vi "_old_Load_SetList_v4.10_DDS.vi"(0 "Path":path) -> (1 "Procedure Name":string="IBS_PICameraTest_29Sep04", 2 "Paramaters":T2={"Master PB Staging List"=[{"Output Bits"=[], "Delay (s)"="", "String"="", "Halt?"=FALSE}, {"Output Bits"=[], "Delay (s)"="", "String"="", "Halt?"=FALSE}, {"Output Bits"=[], "Delay (s)"="", "String"="", "Halt?"=FALSE}, {"Output Bits"=[], "Delay (s)"="", "String"="", "Halt?"=FALSE}, {"Output Bits"=[], "Delay (s)"="", "String"="", "Halt?"=FALSE}, {"Output Bits"=[], "Delay (s)"="", "String"="", "Halt?"=FALSE}, {"Output Bits"=[], "Delay (s)"="", "String"="", "Halt?"=FALSE}, {"Output Bits"=[], "Delay (s)"="", "String"="", "Halt?"=FALSE}, {"Output Bits"=[], "Delay (s)"="", "String"="", "Halt?"=FALSE}, {"Output Bits"=[], "Delay (s)"="", "String"="", "Halt?"=FALSE}, {"Output Bits"=[], "Delay (s)"="", "String"="", "Halt?"=FALSE}, {"Output Bits"=[], "Delay (s)"="", "String"="", "Halt?"=FALSE}, {"Output Bits"=[], "Delay (s)"="", "String"="", "Halt?"=FALSE}, {"Output Bits"=[], "Delay (s)"="", "String"="", "Halt?"=FALSE}, {"Output Bits"=[], "Delay (s)"="", "String"="", "Halt?"=FALSE}, {"Output Bits"=[], "Delay (s)"="", "String"="", "Halt?"=FALSE}, {"Output Bits"=[], "Delay (s)"="", "String"="", "Halt?"=FALSE}, {"Output Bits"=[], "Delay (s)"="", "String"="", "Halt?"=FALSE}, {"Output Bits"=[], "Delay (s)"="", "String"="", "Halt?"=FALSE}, {"Output Bits"=[], "Delay (s)"="", "String"="", "Halt?"=FALSE}, {"Output Bits"=[], "Delay (s)"="", "String"="", "Halt?"=FALSE}, {"Output Bits"=[], "Delay (s)"="", "String"="", "Halt?"=FALSE}, {"Output Bits"=[], "Delay (s)"="", "String"="", "Halt?"=FALSE}, {"Output Bits"=[], "Delay (s)"="", "String"="", "Halt?"=FALSE}, {"Output Bits"=[], "Delay (s)"="", "String"="", "Halt?"=FALSE}, {"Output Bits"=[], "Delay (s)"="", "String"="", "Halt?"=FALSE}, {"Output Bits"=[], "Delay (s)"="", "String"="", "Halt?"=FALSE}, {"Output Bits"=[], "Delay (s)"="", "String"="", "Halt?"=FALSE}, {"Output Bits"=[], "Delay (s)"="", "String"="", "Halt?"=FALSE}, {"Output Bits"=[], "Delay (s)"="", "String"="", "Halt?"=FALSE}, {"Output Bits"=[], "Delay (s)"="", "String"="", "Halt?"=FALSE}, {"Output Bits"=[], "Delay (s)"="", "String"="", "Halt?"=FALSE}, {"Output Bits"=[], "Delay (s)"="", "String"="", "Halt?"=FALSE}, {"Output Bits"=[], "Delay (s)"="", "String"="", "Halt?"=FALSE}, {"Output Bits"=[], "Delay (s)"="", "String"="", "Halt?"=FALSE}, {"Output Bits"=[], "Delay (s)"="", "String"="", "Halt?"=FALSE}, {"Output Bits"=[], "Delay (s)"="", "String"="", "Halt?"=FALSE}, {"Output Bits"=[], "Delay (s)"="", "String"="", "Halt?"=FALSE}, {"Output Bits"=[], "Delay (s)"="", "String"="", "Halt?"=FALSE}, {"Output Bits"=[], "Delay (s)"="", "String"="", "Halt?"=FALSE}, {"Output Bits"=[], "Delay (s)"="", "String"="", "Halt?"=FALSE}, {"Output Bits"=[], "Delay (s)"="", "String"="", "Halt?"=FALSE}, {"Output Bits"=[], "Delay (s)"="", "String"="", "Halt?"=FALSE}, {"Output Bits"=[], "Delay (s)"="", "String"="", "Halt?"=FALSE}], "Slave PB Staging List"=[{"Output Bits"=[], "Delay (s)"="", "String"="", "Halt?"=FALSE}, {"Output Bits"=[], "Delay (s)"="", "String"="", "Halt?"=FALSE}, {"Output Bits"=[], "Delay (s)"="", "String"="", "Halt?"=FALSE}, {"Output Bits"=[], "Delay (s)"="", "String"="", "Halt?"=FALSE}, {"Output Bits"=[], "Delay (s)"="", "String"="", "Halt?"=FALSE}, {"Output Bits"=[], "Delay (s)"="", "String"="", "Halt?"=FALSE}, {"Output Bits"=[], "Delay (s)"="", "String"="", "Halt?"=FALSE}, {"Output Bits"=[], "Delay (s)"="", "String"="", "Halt?"=FALSE}, {"Output Bits"=[], "Delay (s)"="", "String"="", "Halt?"=FALSE}, {"Output Bits"=[], "Delay (s)"="", "String"="", "Halt?"=FALSE}, {"Output Bits"=[], "Delay (s)"="", "String"="", "Halt?"=FALSE}, {"Output Bits"=[], "Delay (s)"="", "String"="", "Halt?"=FALSE}, {"Output Bits"=[], "Delay (s)"="", "String"="", "Halt?"=FALSE}, {"Output Bits"=[], "Delay (s)"="", "String"="", "Halt?"=FALSE}, {"Output Bits"=[], "Delay (s)"="", "String"="", "Halt?"=FALSE}, {"Output Bits"=[], "Delay (s)"="", "String"="", "Halt?"=FALSE}, {"Output Bits"=[], "Delay (s)"="", "String"="", "Halt?"=FALSE}, {"Output Bits"=[], "Delay (s)"="", "String"="", "Halt?"=FALSE}, {"Output Bits"=[], "Delay (s)"="", "String"="", "Halt?"=FALSE}, {"Output Bits"=[], "Delay (s)"="", "String"="", "Halt?"=FALSE}, {"Output Bits"=[], "Delay (s)"="", "String"="", "Halt?"=FALSE}, {"Output Bits"=[], "Delay (s)"="", "String"="", "Halt?"=FALSE}, {"Output Bits"=[], "Delay (s)"="", "String"="", "Halt?"=FALSE}, {"Output Bits"=[], "Delay (s)"="", "String"="", "Halt?"=FALSE}, {"Output Bits"=[], "Delay (s)"="", "String"="", "Halt?"=FALSE}, {"Output Bits"=[], "Delay (s)"="", "String"="", "Halt?"=FALSE}, {"Output Bits"=[], "Delay (s)"="", "String"="", "Halt?"=FALSE}, {"Output Bits"=[], "Delay (s)"="", "String"="", "Halt?"=FALSE}, {"Output Bits"=[], "Delay (s)"="", "String"="", "Halt?"=FALSE}, {"Output Bits"=[], "Delay (s)"="", "String"="", "Halt?"=FALSE}, {"Output Bits"=[], "Delay (s)"="", "String"="", "Halt?"=FALSE}, {"Output Bits"=[], "Delay (s)"="", "String"="", "Halt?"=FALSE}, {"Output Bits"=[], "Delay (s)"="", "String"="", "Halt?"=FALSE}, {"Output Bits"=[], "Delay (s)"="", "String"="", "Halt?"=FALSE}, {"Output Bits"=[], "Delay (s)"="", "String"="", "Halt?"=FALSE}, {"Output Bits"=[], "Delay (s)"="", "String"="", "Halt?"=FALSE}, {"Output Bits"=[], "Delay (s)"="", "String"="", "Halt?"=FALSE}, {"Output Bits"=[], "Delay (s)"="", "String"="", "Halt?"=FALSE}, {"Output Bits"=[], "Delay (s)"="", "String"="", "Halt?"=FALSE}, {"Output Bits"=[], "Delay (s)"="", "String"="", "Halt?"=FALSE}, {"Output Bits"=[], "Delay (s)"="", "String"="", "Halt?"=FALSE}, {"Output Bits"=[], "Delay (s)"="", "String"="", "Halt?"=FALSE}, {"Output Bits"=[], "Delay (s)"="", "String"="", "Halt?"=FALSE}, {"Output Bits"=[], "Delay (s)"="", "String"="", "Halt?"=FALSE}], "Novatech Ramps"=[{"Ramp Channels"=[], "2 Freq. [MHz]"="", "2 Power [dBm]"="", "3 Freq. [MHz]"="", "3 Power [dBm]"="", "Serial Port"=""}, {"Ramp Channels"=[], "2 Freq. [MHz]"="", "2 Power [dBm]"="", "3 Freq. [MHz]"="", "3 Power [dBm]"="", "Serial Port"=""}, {"Ramp Channels"=[], "2 Freq. [MHz]"="", "2 Power [dBm]"="", "3 Freq. [MHz]"="", "3 Power [dBm]"="", "Serial Port"=""}, {"Ramp Channels"=[], "2 Freq. [MHz]"="", "2 Power [dBm]"="", "3 Freq. [MHz]"="", "3 Power [dBm]"="", "Serial Port"=""}, {"Ramp Channels"=[], "2 Freq. [MHz]"="", "2 Power [dBm]"="", "3 Freq. [MHz]"="", "3 Power [dBm]"="", "Serial Port"=""}, {"Ramp Channels"=[], "2 Freq. [MHz]"="", "2 Power [dBm]"="", "3 Freq. [MHz]"="", "3 Power [dBm]"="", "Serial Port"=""}, {"Ramp Channels"=[], "2 Freq. [MHz]"="", "2 Power [dBm]"="", "3 Freq. [MHz]"="", "3 Power [dBm]"="", "Serial Port"=""}], "Sequencing Info"=[{"Start"=0.0, "End"=2.11, "Sequenced Data"=[], "Inform\nIgor?"=FALSE, "Computed Step Size"=0.0, "Procedure Variable"="", "Default"=2.11, "Steps"=0}], "SRS Ramps"=[{"lattice ramp"=[{"dt"="", "formula"=""}, {"dt"="", "formula"=""}, {"dt"="", "formula"=""}], "Output"=[{"Time Values"=[0.0, 0.002, 0.004, 0.006, 0.008, 0.01, 0.012, 0.014, 0.016, 0.018000000000000002, 0.02, 0.022, 0.024, 0.026000000000000002, 0.028, 0.03, 0.032, 0.034, 0.036000000000000004, 0.038, 0.04, 0.042, 0.044, 0.046, 0.048, 0.05, 0.052000000000000005, 0.054, 0.056, 0.058, 0.06, 0.062, 0.064, 0.066, 0.068, 0.07, 0.07200000000000001, 0.074, 0.076, 0.078, 0.08, 0.082, 0.084, 0.08600000000000001, 0.088, 0.09, 0.092, 0.094, 0.096, 0.098, 0.1, 0.10200000000000001, 0.10400000000000001, 0.106, 0.108, 0.11, 0.112, 0.114, 0.116, 0.11800000000000001, 0.12, 0.122, 0.124, 0.126, 0.128, 0.13, 0.132, 0.134, 0.136, 0.138, 0.14, 0.14200000000000002, 0.14400000000000002, 0.146, 0.148, 0.15, 0.152, 0.154, 0.156, 0.158, 0.16, 0.162, 0.164, 0.166, 0.168, 0.17, 0.17200000000000001, 0.17400000000000002, 0.176, 0.178, 0.18, 0.182, 0.184, 0.186, 0.188, 0.19, 0.192, 0.194, 0.196, 0.198, 0.2, 0.6000000000000001, 0.6000000000000001, 0.6002000000000001, 0.6004, 0.6006000000000001, 0.6008000000000001, 0.6010000000000001, 0.6012000000000001, 0.6014, 0.6016000000000001, 0.6018000000000001, 0.6020000000000001, 0.6022000000000001, 0.6024, 0.6026000000000001, 0.6028000000000001, 0.6030000000000001, 0.6032000000000001, 0.6034, 0.6036000000000001, 0.6038000000000001, 0.6040000000000001, 0.6042000000000001, 0.6044, 0.6046000000000001, 0.6048000000000001, 0.6050000000000001, 0.6052000000000001, 0.6054, 0.6056000000000001, 0.6058000000000001, 0.6060000000000001, 0.6062000000000001, 0.6064, 0.6066000000000001, 0.6068000000000001, 0.6070000000000001, 0.6072000000000001, 0.6074, 0.6076000000000001, 0.6078000000000001, 0.6080000000000001, 0.6082000000000001, 0.6084, 0.6086000000000001, 0.6088000000000001, 0.6090000000000001, 0.6092000000000001, 0.6094, 0.6096000000000001, 0.6098000000000001, 0.6100000000000001, 0.6102000000000001, 0.6104, 0.6106000000000001, 0.6108000000000001, 0.6110000000000001, 0.6112000000000001, 0.6114, 0.6116000000000001, 0.6118000000000001, 0.6120000000000001, 0.6122000000000001, 0.6124, 0.6126, 0.6128000000000001, 0.6130000000000001, 0.6132000000000001, 0.6134000000000001, 0.6136000000000001, 0.6138000000000001, 0.6140000000000001, 0.6142000000000001, 0.6144000000000001, 0.6146, 0.6148000000000001, 0.6150000000000001, 0.6152000000000001, 0.6154000000000001, 0.6156, 0.6158000000000001, 0.6160000000000001, 0.6162000000000001, 0.6164000000000001, 0.6166, 0.6168000000000001, 0.6170000000000001, 0.6172000000000001, 0.6174000000000001, 0.6176, 0.6178000000000001, 0.6180000000000001, 0.6182000000000001, 0.6184000000000001, 0.6186, 0.6188000000000001, 0.6190000000000001, 0.6192000000000001, 0.6194000000000001, 0.6196, 0.6198000000000001, 0.6200000000000001, 0.6202000000000001, 0.6212000000000001], array[205 elements]}, {"Time Values"=[0.0, 0.002, 0.004, 0.006, 0.008, 0.01, 0.012, 0.014, 0.016, 0.018000000000000002, 0.02, 0.022, 0.024, 0.026000000000000002, 0.028, 0.03, 0.032, 0.034, 0.036000000000000004, 0.038, 0.04, 0.042, 0.044, 0.046, 0.048, 0.05, 0.052000000000000005, 0.054, 0.056, 0.058, 0.06, 0.062, 0.064, 0.066, 0.068, 0.07, 0.07200000000000001, 0.074, 0.076, 0.078, 0.08, 0.082, 0.084, 0.08600000000000001, 0.088, 0.09, 0.092, 0.094, 0.096, 0.098, 0.1, 0.10200000000000001, 0.10400000000000001, 0.106, 0.108, 0.11, 0.112, 0.114, 0.116, 0.11800000000000001, 0.12, 0.122, 0.124, 0.126, 0.128, 0.13, 0.132, 0.134, 0.136, 0.138, 0.14, 0.14200000000000002, 0.14400000000000002, 0.146, 0.148, 0.15, 0.152, 0.154, 0.156, 0.158, 0.16, 0.162, 0.164, 0.166, 0.168, 0.17, 0.17200000000000001, 0.17400000000000002, 0.176, 0.178, 0.18, 0.182, 0.184, 0.186, 0.188, 0.19, 0.192, 0.194, 0.196, 0.198, 0.2, 0.6000000000000001, 0.6000000000000001, 0.6002000000000001, 0.6004, 0.6006000000000001, 0.6008000000000001, 0.6010000000000001, 0.6012000000000001, 0.6014, 0.6016000000000001, 0.6018000000000001, 0.6020000000000001, 0.6022000000000001, 0.6024, 0.6026000000000001, 0.6028000000000001, 0.6030000000000001, 0.6032000000000001, 0.6034, 0.6036000000000001, 0.6038000000000001, 0.6040000000000001, 0.6042000000000001, 0.6044, 0.6046000000000001, 0.6048000000000001, 0.6050000000000001, 0.6052000000000001, 0.6054, 0.6056000000000001, 0.6058000000000001, 0.6060000000000001, 0.6062000000000001, 0.6064, 0.6066000000000001, 0.6068000000000001, 0.6070000000000001, 0.6072000000000001, 0.6074, 0.6076000000000001, 0.6078000000000001, 0.6080000000000001, 0.6082000000000001, 0.6084, 0.6086000000000001, 0.6088000000000001, 0.6090000000000001, 0.6092000000000001, 0.6094, 0.6096000000000001, 0.6098000000000001, 0.6100000000000001, 0.6102000000000001, 0.6104, 0.6106000000000001, 0.6108000000000001, 0.6110000000000001, 0.6112000000000001, 0.6114, 0.6116000000000001, 0.6118000000000001, 0.6120000000000001, 0.6122000000000001, 0.6124, 0.6126, 0.6128000000000001, 0.6130000000000001, 0.6132000000000001, 0.6134000000000001, 0.6136000000000001, 0.6138000000000001, 0.6140000000000001, 0.6142000000000001, 0.6144000000000001, 0.6146, 0.6148000000000001, 0.6150000000000001, 0.6152000000000001, 0.6154000000000001, 0.6156, 0.6158000000000001, 0.6160000000000001, 0.6162000000000001, 0.6164000000000001, 0.6166, 0.6168000000000001, 0.6170000000000001, 0.6172000000000001, 0.6174000000000001, 0.6176, 0.6178000000000001, 0.6180000000000001, 0.6182000000000001, 0.6184000000000001, 0.6186, 0.6188000000000001, 0.6190000000000001, 0.6192000000000001, 0.6194000000000001, 0.6196, 0.6198000000000001, 0.6200000000000001, 0.6202000000000001, 0.6212000000000001], array[205 elements]}], "SRS Selection"=enum."1550 Vertical"}, {"lattice ramp"=[{"dt"="", "formula"=""}], "Output"=[{"Time Values"=[0.0, 0.002, 0.004, 0.006, 0.008, 0.01, 0.012, 0.014, 0.016, 0.018000000000000002, 0.02, 0.022, 0.024, 0.026000000000000002, 0.028, 0.03, 0.032, 0.034, 0.036000000000000004, 0.038, 0.04, 0.042, 0.044, 0.046, 0.048, 0.05, 0.052000000000000005, 0.054, 0.056, 0.058, 0.06, 0.062, 0.064, 0.066, 0.068, 0.07, 0.07200000000000001, 0.074, 0.076, 0.078, 0.08, 0.082, 0.084, 0.08600000000000001, 0.088, 0.09, 0.092, 0.094, 0.096, 0.098, 0.1, 0.10200000000000001, 0.10400000000000001, 0.106, 0.108, 0.11, 0.112, 0.114, 0.116, 0.11800000000000001, 0.12, 0.122, 0.124, 0.126, 0.128, 0.13, 0.132, 0.134, 0.136, 0.138, 0.14, 0.14200000000000002, 0.14400000000000002, 0.146, 0.148, 0.15, 0.152, 0.154, 0.156, 0.158, 0.16, 0.162, 0.164, 0.166, 0.168, 0.17, 0.17200000000000001, 0.17400000000000002, 0.176, 0.178, 0.18, 0.182, 0.184, 0.186, 0.188, 0.19, 0.192, 0.194, 0.196, 0.198, 0.2, 0.6000000000000001, 0.6000000000000001, 0.6002000000000001, 0.6004, 0.6006000000000001, 0.6008000000000001, 0.6010000000000001, 0.6012000000000001, 0.6014, 0.6016000000000001, 0.6018000000000001, 0.6020000000000001, 0.6022000000000001, 0.6024, 0.6026000000000001, 0.6028000000000001, 0.6030000000000001, 0.6032000000000001, 0.6034, 0.6036000000000001, 0.6038000000000001, 0.6040000000000001, 0.6042000000000001, 0.6044, 0.6046000000000001, 0.6048000000000001, 0.6050000000000001, 0.6052000000000001, 0.6054, 0.6056000000000001, 0.6058000000000001, 0.6060000000000001, 0.6062000000000001, 0.6064, 0.6066000000000001, 0.6068000000000001, 0.6070000000000001, 0.6072000000000001, 0.6074, 0.6076000000000001, 0.6078000000000001, 0.6080000000000001, 0.6082000000000001, 0.6084, 0.6086000000000001, 0.6088000000000001, 0.6090000000000001, 0.6092000000000001, 0.6094, 0.6096000000000001, 0.6098000000000001, 0.6100000000000001, 0.6102000000000001, 0.6104, 0.6106000000000001, 0.6108000000000001, 0.6110000000000001, 0.6112000000000001, 0.6114, 0.6116000000000001, 0.6118000000000001, 0.6120000000000001, 0.6122000000000001, 0.6124, 0.6126, 0.6128000000000001, 0.6130000000000001, 0.6132000000000001, 0.6134000000000001, 0.6136000000000001, 0.6138000000000001, 0.6140000000000001, 0.6142000000000001, 0.6144000000000001, 0.6146, 0.6148000000000001, 0.6150000000000001, 0.6152000000000001, 0.6154000000000001, 0.6156, 0.6158000000000001, 0.6160000000000001, 0.6162000000000001, 0.6164000000000001, 0.6166, 0.6168000000000001, 0.6170000000000001, 0.6172000000000001, 0.6174000000000001, 0.6176, 0.6178000000000001, 0.6180000000000001, 0.6182000000000001, 0.6184000000000001, 0.6186, 0.6188000000000001, 0.6190000000000001, 0.6192000000000001, 0.6194000000000001, 0.6196, 0.6198000000000001, 0.6200000000000001, 0.6202000000000001, 0.6212000000000001], array[205 elements]}, {"Time Values"=[0.0, 0.002, 0.004, 0.006, 0.008, 0.01, 0.012, 0.014, 0.016, 0.018000000000000002, 0.02, 0.022, 0.024, 0.026000000000000002, 0.028, 0.03, 0.032, 0.034, 0.036000000000000004, 0.038, 0.04, 0.042, 0.044, 0.046, 0.048, 0.05, 0.052000000000000005, 0.054, 0.056, 0.058, 0.06, 0.062, 0.064, 0.066, 0.068, 0.07, 0.07200000000000001, 0.074, 0.076, 0.078, 0.08, 0.082, 0.084, 0.08600000000000001, 0.088, 0.09, 0.092, 0.094, 0.096, 0.098, 0.1, 0.10200000000000001, 0.10400000000000001, 0.106, 0.108, 0.11, 0.112, 0.114, 0.116, 0.11800000000000001, 0.12, 0.122, 0.124, 0.126, 0.128, 0.13, 0.132, 0.134, 0.136, 0.138, 0.14, 0.14200000000000002, 0.14400000000000002, 0.146, 0.148, 0.15, 0.152, 0.154, 0.156, 0.158, 0.16, 0.162, 0.164, 0.166, 0.168, 0.17, 0.17200000000000001, 0.17400000000000002, 0.176, 0.178, 0.18, 0.182, 0.184, 0.186, 0.188, 0.19, 0.192, 0.194, 0.196, 0.198, 0.2, 0.6000000000000001, 0.6000000000000001, 0.6002000000000001, 0.6004, 0.6006000000000001, 0.6008000000000001, 0.6010000000000001, 0.6012000000000001, 0.6014, 0.6016000000000001, 0.6018000000000001, 0.6020000000000001, 0.6022000000000001, 0.6024, 0.6026000000000001, 0.6028000000000001, 0.6030000000000001, 0.6032000000000001, 0.6034, 0.6036000000000001, 0.6038000000000001, 0.6040000000000001, 0.6042000000000001, 0.6044, 0.6046000000000001, 0.6048000000000001, 0.6050000000000001, 0.6052000000000001, 0.6054, 0.6056000000000001, 0.6058000000000001, 0.6060000000000001, 0.6062000000000001, 0.6064, 0.6066000000000001, 0.6068000000000001, 0.6070000000000001, 0.6072000000000001, 0.6074, 0.6076000000000001, 0.6078000000000001, 0.6080000000000001, 0.6082000000000001, 0.6084, 0.6086000000000001, 0.6088000000000001, 0.6090000000000001, 0.6092000000000001, 0.6094, 0.6096000000000001, 0.6098000000000001, 0.6100000000000001, 0.6102000000000001, 0.6104, 0.6106000000000001, 0.6108000000000001, 0.6110000000000001, 0.6112000000000001, 0.6114, 0.6116000000000001, 0.6118000000000001, 0.6120000000000001, 0.6122000000000001, 0.6124, 0.6126, 0.6128000000000001, 0.6130000000000001, 0.6132000000000001, 0.6134000000000001, 0.6136000000000001, 0.6138000000000001, 0.6140000000000001, 0.6142000000000001, 0.6144000000000001, 0.6146, 0.6148000000000001, 0.6150000000000001, 0.6152000000000001, 0.6154000000000001, 0.6156, 0.6158000000000001, 0.6160000000000001, 0.6162000000000001, 0.6164000000000001, 0.6166, 0.6168000000000001, 0.6170000000000001, 0.6172000000000001, 0.6174000000000001, 0.6176, 0.6178000000000001, 0.6180000000000001, 0.6182000000000001, 0.6184000000000001, 0.6186, 0.6188000000000001, 0.6190000000000001, 0.6192000000000001, 0.6194000000000001, 0.6196, 0.6198000000000001, 0.6200000000000001, 0.6202000000000001, 0.6212000000000001], array[205 elements]}], "SRS Selection"=enum."1550 Vertical"}], "Master AO Ramp List"=[{"Ramp index"=10, "Ramp time [s]"="", "Step size [s]"=1000.0, "Ramp Array"=[], "Output Bits"=[]}, {"Ramp index"=10, "Ramp time [s]"="", "Step size [s]"=1000.0, "Ramp Array"=[], "Output Bits"=[]}], "Slave AO Ramp List"=[{"Ramp index"=10, "Ramp time [s]"="", "Step size [s]"=1000.0, "Ramp Array"=[], "Output Bits"=[]}, {"Ramp index"=10, "Ramp time [s]"="", "Step size [s]"=1000.0, "Ramp Array"=[], "Output Bits"=[]}], "Master Novatech Ramp List"=[], "Static Variables"=[], "DDS Ramp List"=[]} {"Sequencing Info"."Steps" min=2; "Sequencing Info"."Default" format="%#.7p"; "Sequencing Info"."Computed Step Size" format="%#.7p"; "Sequencing Info"."Sequenced Data" format="%.2e"; "Sequencing Info"."End" format="%#.7p"; "Sequencing Info"."Start" format="%#.7p"})   [LabVIEW 2013]
uses:
  TypeDefs/Active procedure variables.ctl
panel:
  out "Array":errorcluster[](array[cluster])
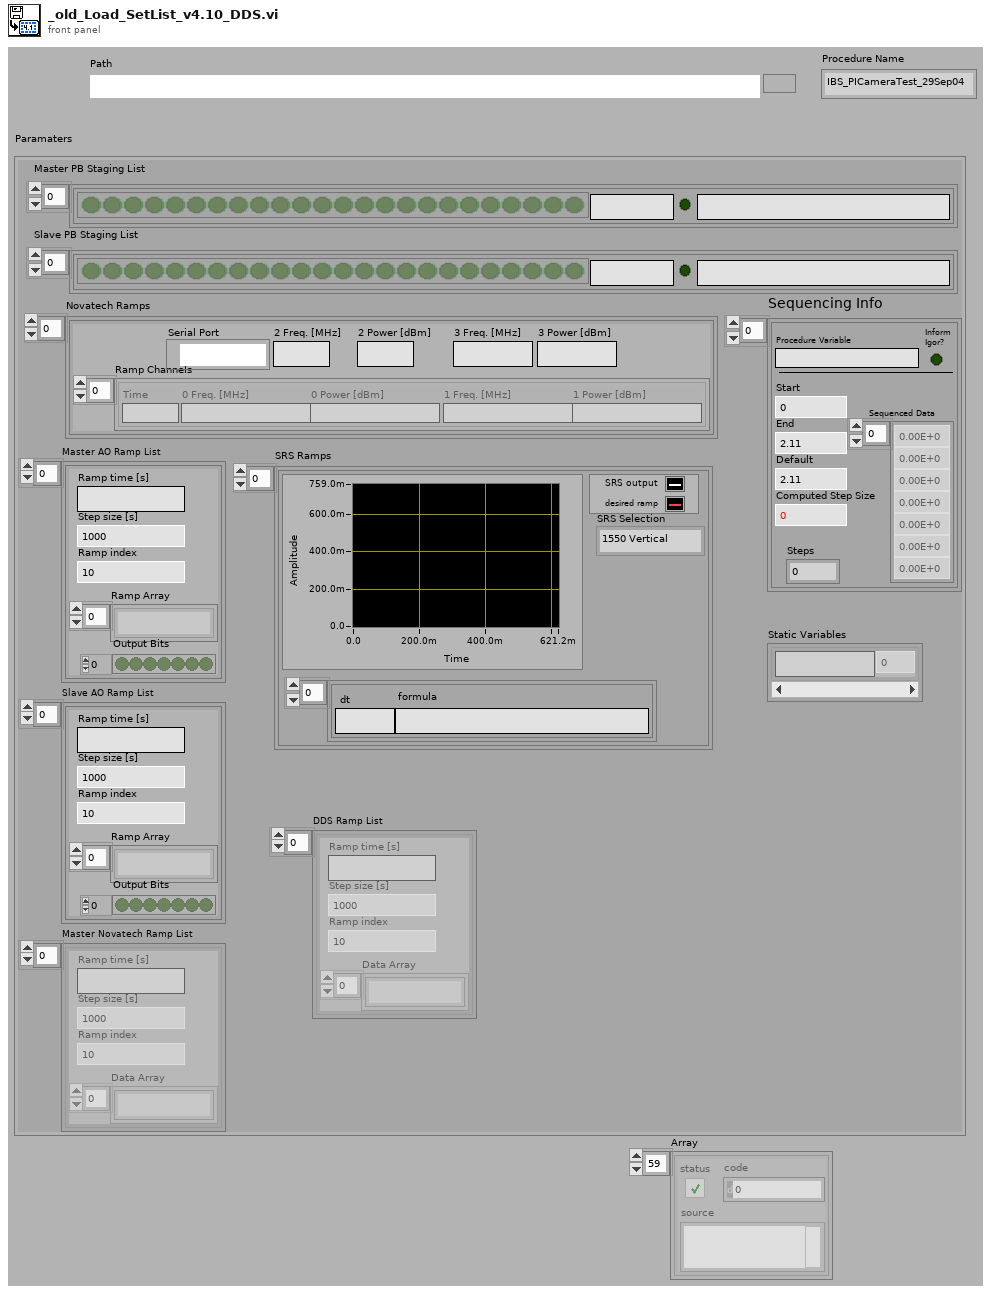
[diagram p1: front panel]
types:
  T1 = typedef "Active procedure variables.ctl" = cluster{"Procedure variable":string, "Value":dbl}
  T2 = cluster{"Master PB Staging List":cluster{"Output Bits":bool[], "Delay (s)":string, "String":string, "Halt?":bool}[], "Slave PB Staging List":cluster{"Output Bits":bool[], "Delay (s)":string, "String":string, "Halt?":bool}[], "Novatech Ramps":cluster{"Ramp Channels":cluster{"Time":string, "0 Freq. [MHz]":string, "0 Power [dBm]":string, "1 Freq. [MHz]":string, "1 Power [dBm]":string}[], "2 Freq. [MHz]":string, "2 Power [dBm]":string, "3 Freq. [MHz]":string, "3 Power [dBm]":string, "Serial Port":refnum<visa-resource-name>}[], "Sequencing Info":cluster{"Start":dbl, "End":dbl, "Sequenced Data":dbl[], "Inform\nIgor?":bool, "Computed Step Size":dbl, "Procedure Variable":string, "Default":dbl, "Steps":i32}[], "SRS Ramps":cluster{"lattice ramp":cluster{"dt":string, "formula":string}[], "Output":cluster{"Time Values":dbl[], dbl[]}[], "SRS Selection":enum16{"1550 Vertical", "Bragg Agilent", "Bragg PTS", "Acc. Intensity"}}[], "Master AO Ramp List":cluster{"Ramp index":u32, "Ramp time [s]":string, "Step size [s]":dbl, "Ramp Array":string[], "Output Bits":bool[]}[], "Slave AO Ramp List":cluster{"Ramp index":u32, "Ramp time [s]":string, "Step size [s]":dbl, "Ramp Array":string[], "Output Bits":bool[]}[], "Master Novatech Ramp List":cluster{"Ramp index":u32, "Ramp time [s]":string, "Step size [s]":dbl, "Data Array":string[]}[], "Static Variables":T1[], "DDS Ramp List":cluster{"Ramp index":u32, "Ramp time [s]":string, "Step size [s]":dbl, "Data Array":string[]}[]}
  T3 = cluster{"Output Bits":bool[], "Delay (s)":string, "String":string, "Halt?":bool}[]
  T4 = cluster{"Ramp index":u32, "Ramp time [s]":string, "Step size [s]":dbl, "Ramp Array":string[], "Output Bits":bool[]}[]
  T5 = cluster{"Ramp index":u32, "Ramp time [s]":string, "Step size [s]":dbl, "Data Array":string[]}[]
  T6 = cluster{"Ramp Channels":cluster{"Time":string, "0 Freq. [MHz]":string, "0 Power [dBm]":string, "1 Freq. [MHz]":string, "1 Power [dBm]":string}[], "2 Freq. [MHz]":string, "2 Power [dBm]":string, "3 Freq. [MHz]":string, "3 Power [dBm]":string, "Serial Port":refnum<visa-resource-name>}[]
  T7 = cluster{"Start":dbl, "End":dbl, "Sequenced Data":dbl[], "Inform\nIgor?":bool, "Computed Step Size":dbl, "Procedure Variable":string, "Default":dbl, "Steps":i32}[]
  T8 = cluster{"lattice ramp":cluster{"dt":string, "formula":string}[], "Output":cluster{"Time Values":dbl[], dbl[]}[], "SRS Selection":enum16{"1550 Vertical", "Bragg Agilent", "Bragg PTS", "Acc. Intensity"}}[]
  T9 = cluster{"Start":dbl, "End":dbl, "Sequenced Data":dbl[], "Inform\nIgor?":bool, "Computed Step Size":dbl, "Procedure Variable":string, "Default":dbl}
  T10 = cluster{"Ramp index":u32, "Ramp time [s]":string, "Step size [s]":dbl, "Ramp Array":string[], "Output Bits":bool[]}
  T11 = cluster{"Ramp index":u32, "Ramp time [s]":string, "Step size [s]":dbl, "Data Array":string[]}
  T12 = cluster{"Output Bits":bool[], "Delay (s)":string, "String":string, "Halt?":bool}
  T13 = cluster{"Ramp Channels":cluster{"Time":string, "0 Freq. [MHz]":string, "0 Power [dBm]":string, "1 Freq. [MHz]":string, "1 Power [dBm]":string}[], "2 Freq. [MHz]":string, "2 Power [dBm]":string, "3 Freq. [MHz]":string, "3 Power [dBm]":string, "Serial Port":refnum<visa-resource-name>}
  T14 = cluster{"Start":dbl, "End":dbl, "Sequenced Data":dbl[], "Inform\nIgor?":bool, "Computed Step Size":dbl, "Procedure Variable":string, "Default":dbl, "Steps":i32}
  T15 = cluster{"lattice ramp":cluster{"dt":string, "formula":string}[], "Output":cluster{"Time Values":dbl[], dbl[]}[], "SRS Selection":enum16{"1550 Vertical", "Bragg Agilent", "Bragg PTS", "Acc. Intensity"}}
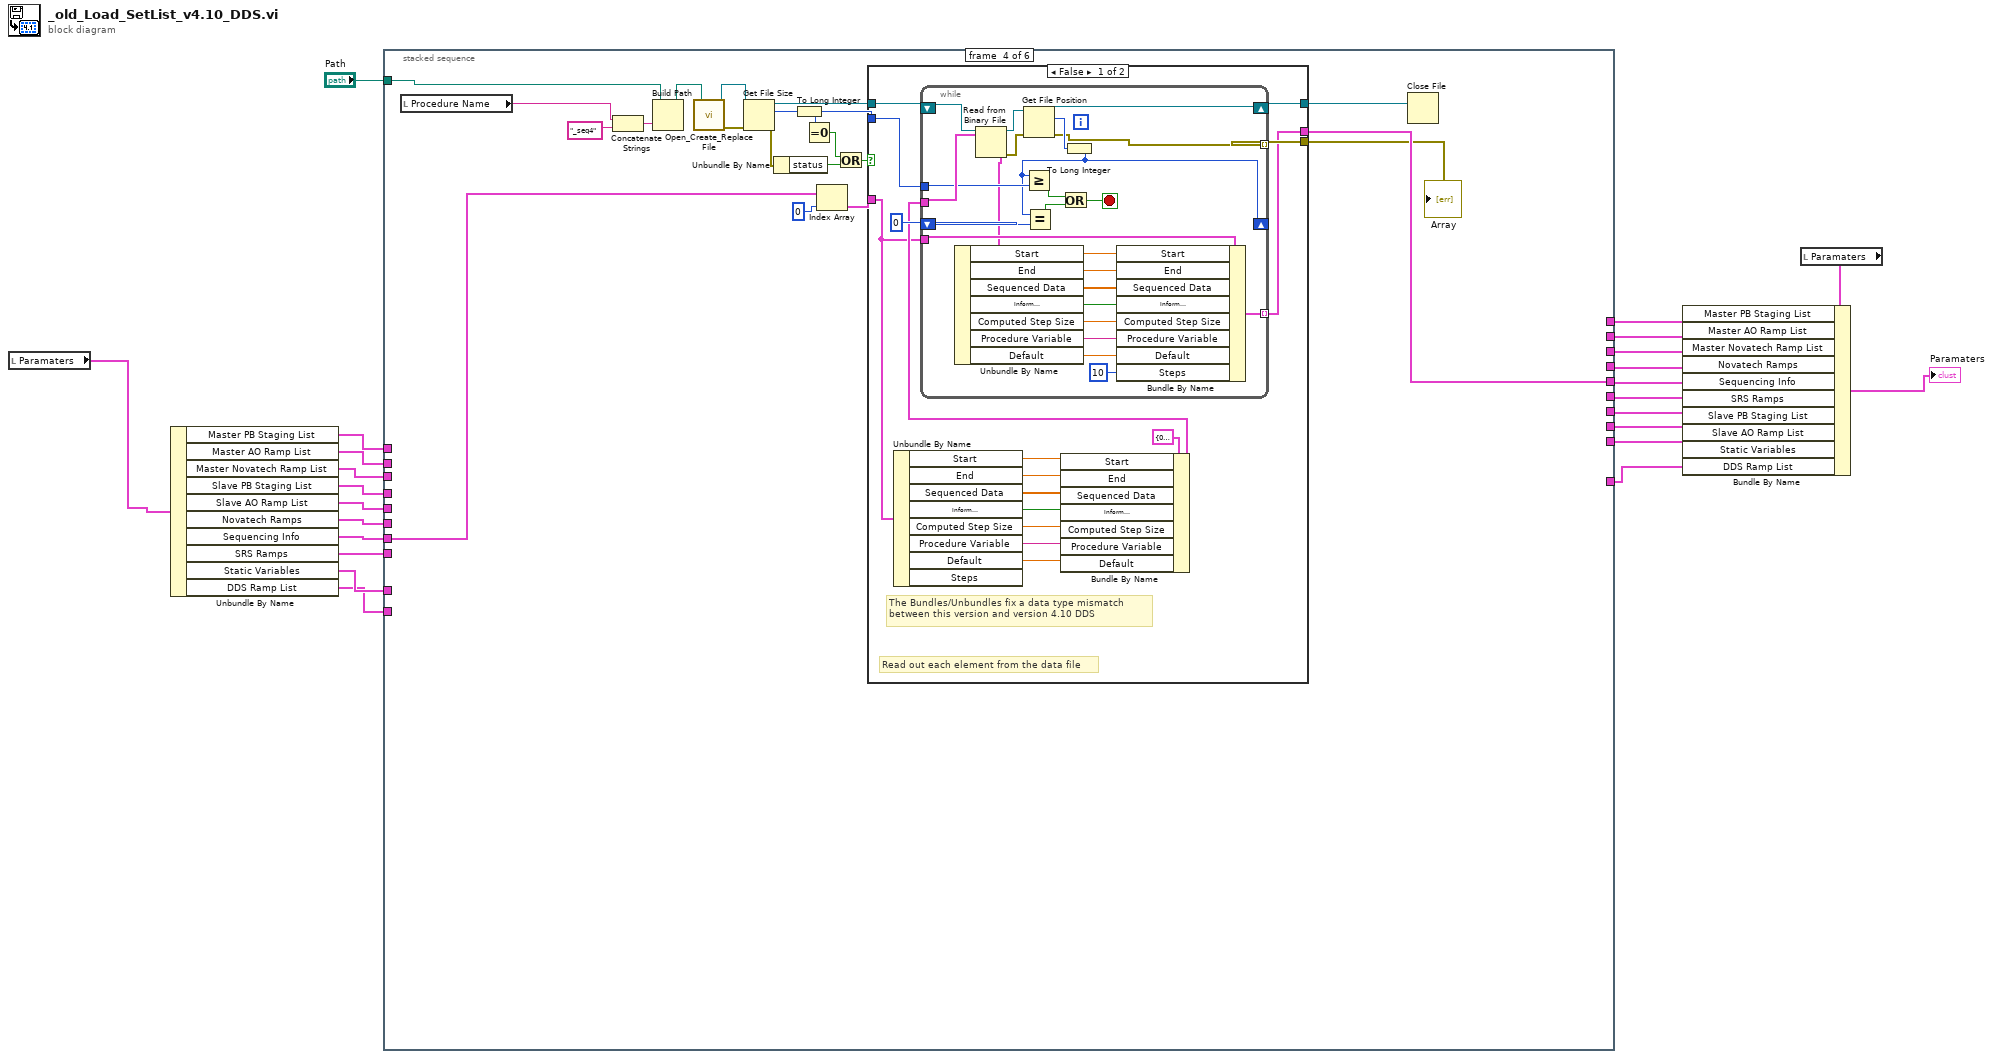
[diagram p0: block diagram]
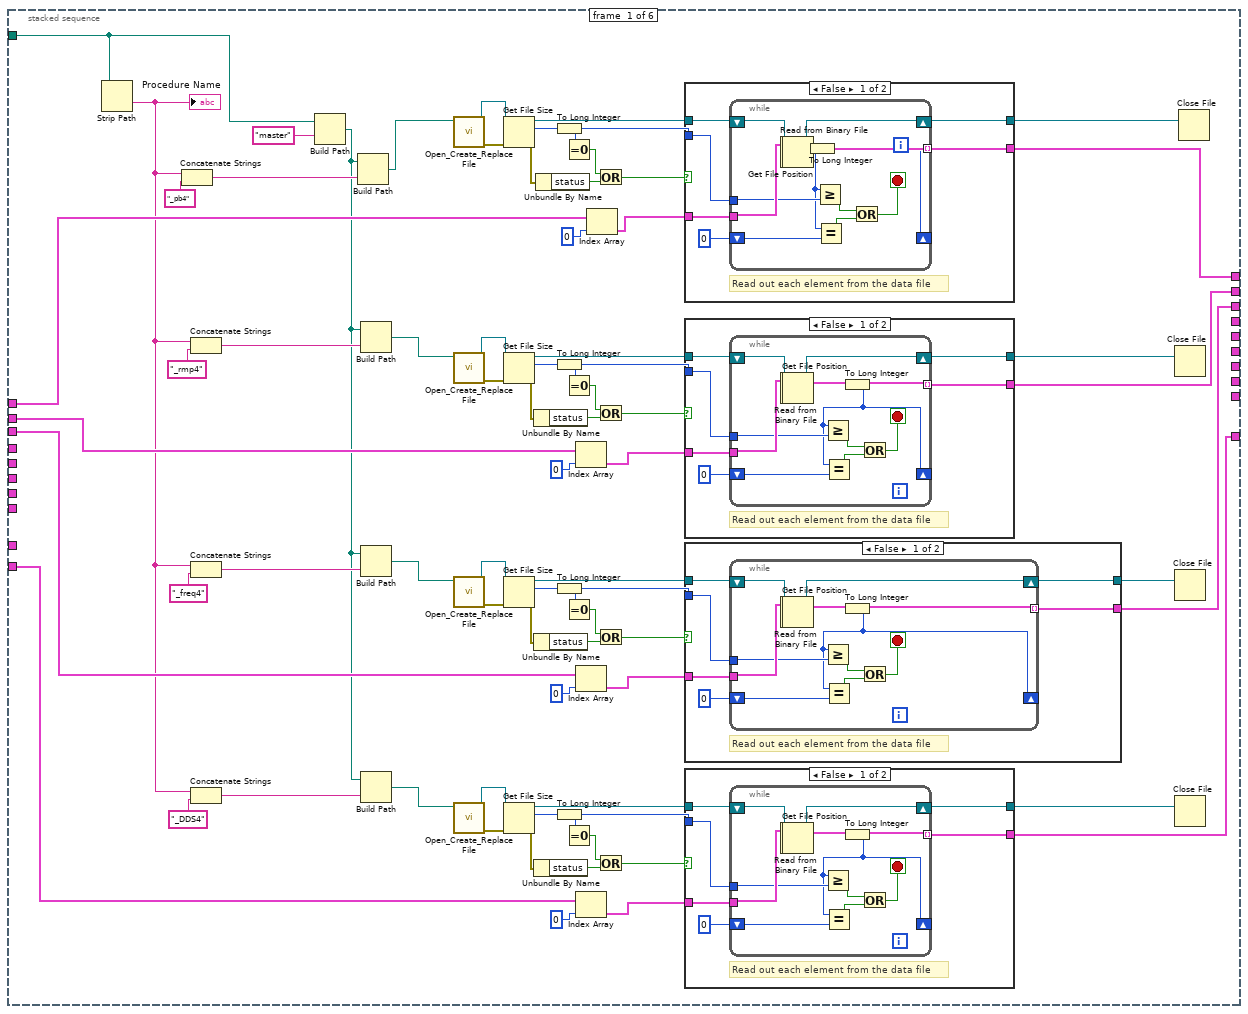
[diagram p2: hidden frame]
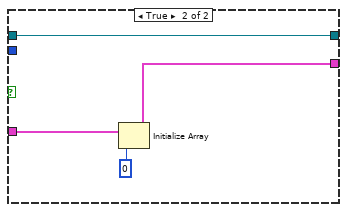
[diagram p3: hidden frame]
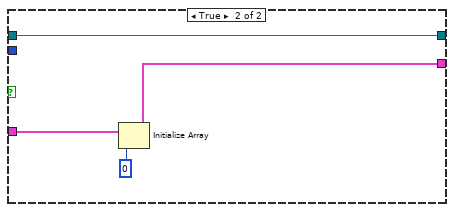
[diagram p4: hidden frame]
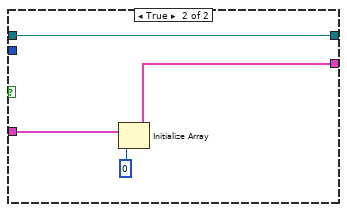
[diagram p5: hidden frame]
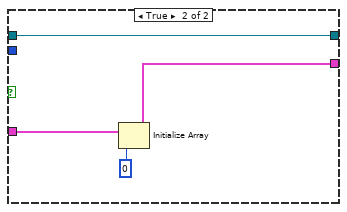
[diagram p6: hidden frame]
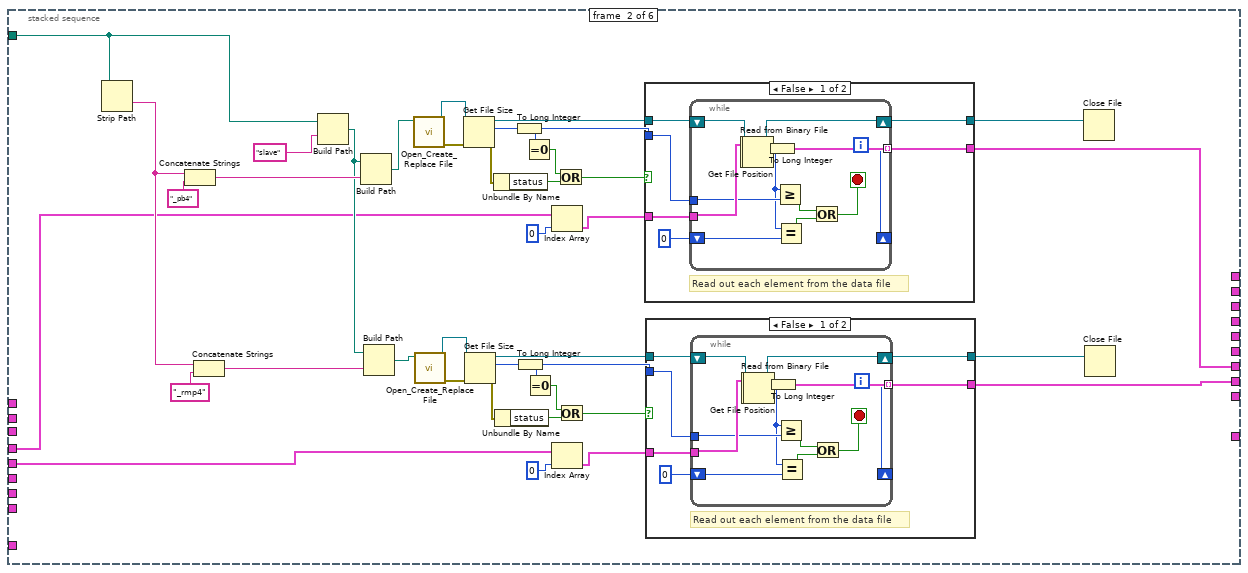
[diagram p7: hidden frame]
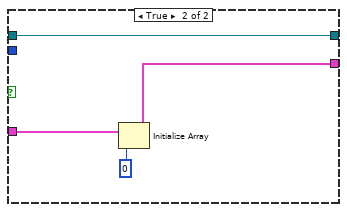
[diagram p8: hidden frame]
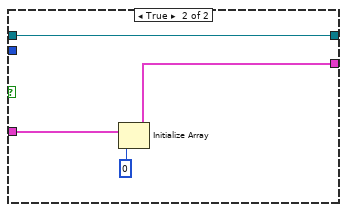
[diagram p9: hidden frame]
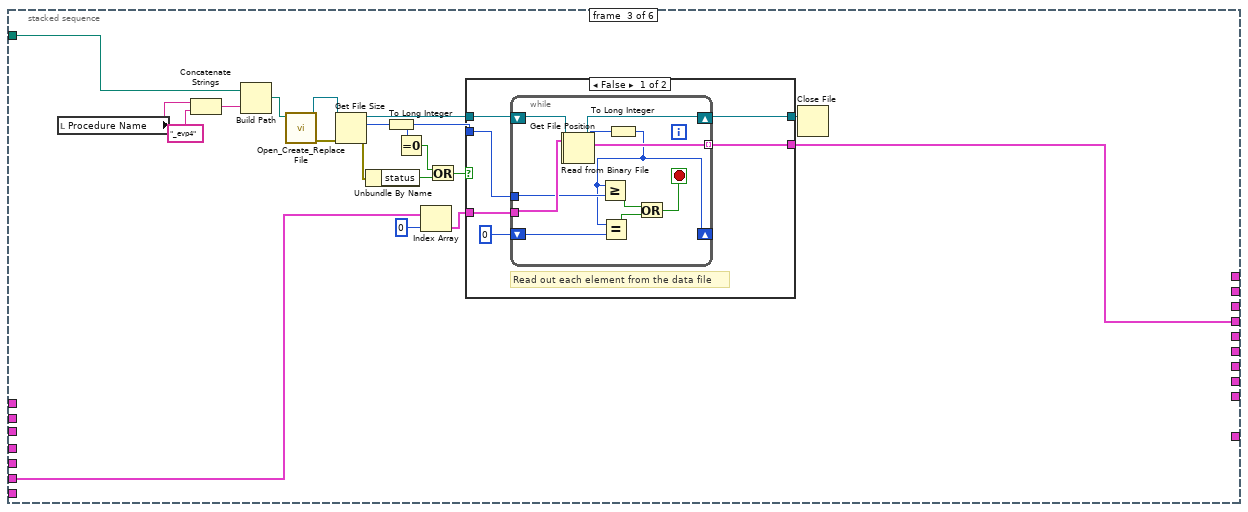
[diagram p10: hidden frame]
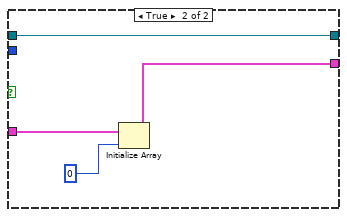
[diagram p11: hidden frame]
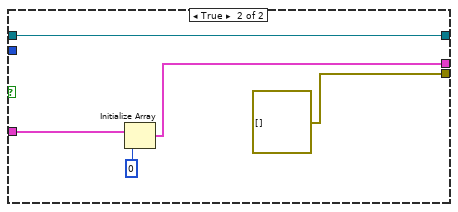
[diagram p12: hidden frame]
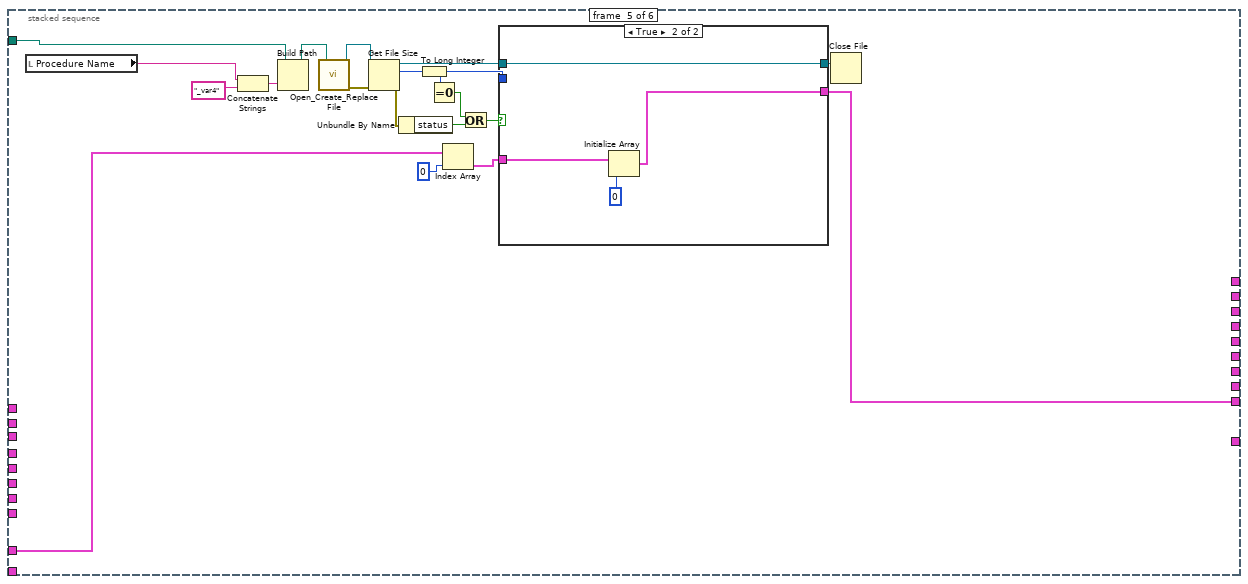
[diagram p13: hidden frame]
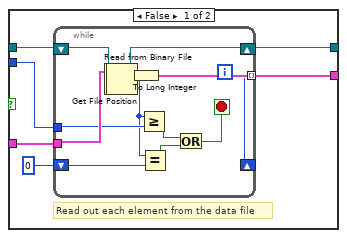
[diagram p14: hidden frame]
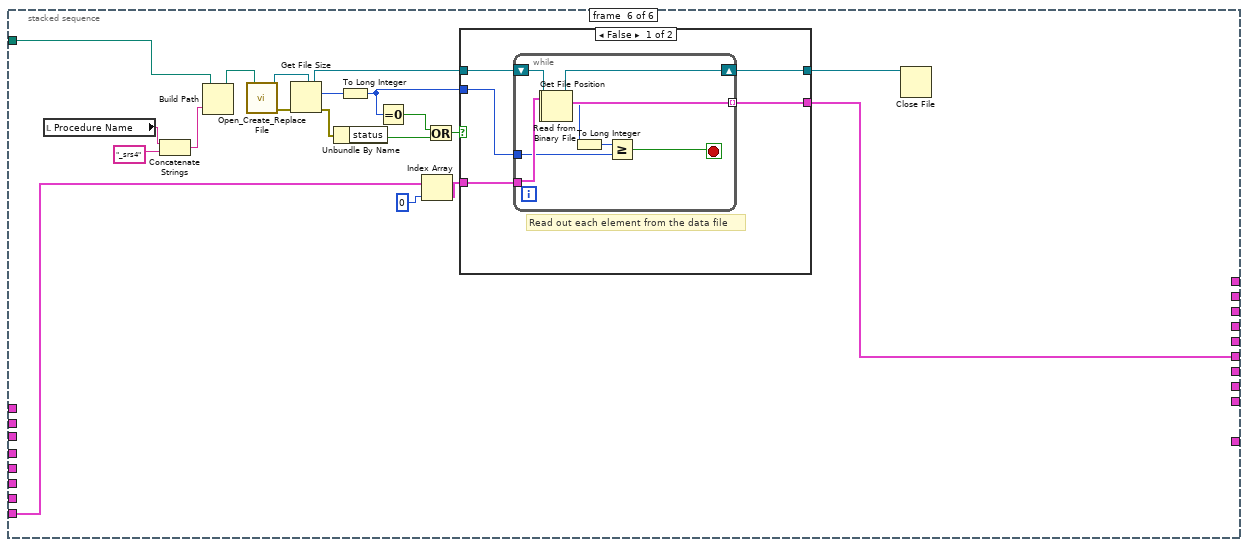
[diagram p15: hidden frame]
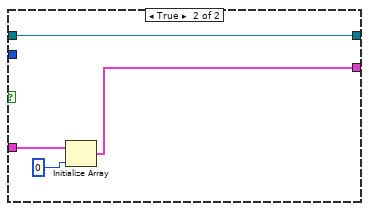
[diagram p16: hidden frame]
diagram:
  n1 = local read "Paramaters"() -> (w1:T2)
  n2 = Unbundle By Name(w1) -> ("Master PB Staging List"=w23:T3, "Master AO Ramp List"=w22:T4, "Master Novatech Ramp List"=w7:T5, "Slave PB Staging List"=w21:T3, "Slave AO Ramp List"=w20:T4, "Novatech Ramps"=w19:T6, "Sequencing Info"=w18:T7, "SRS Ramps"=w17:T8, "Static Variables"=w6:T1[], "DDS Ramp List"=w4:T5)
  n3 = stacked-sequence {
    tunnel: [_ _ _ _ _ w434] -> w9
    tunnel: [_ _ _ w327 _ _] -> w10
    tunnel: w23 -> [w65 _ _ _ _ _]
    tunnel: w22 -> [w61 _ _ _ _ _]
    tunnel: w21 -> [_ w192 _ _ _ _]
    tunnel: w20 -> [_ w189 _ _ _ _]
    tunnel: w19 -> [_ _ w278 _ _ _]
    tunnel: w18 -> [_ _ _ w316 _ _]
    tunnel: w17 -> [_ _ _ _ _ w422]
    tunnel: [w81 _ _ _ _ _] -> w16
    tunnel: "Path" -> [w70 w209 w276 w319 w384 w425]
    tunnel: [w69 _ _ _ _ _] -> w14
    tunnel: [_ _ w273 _ _ _] -> w11
    tunnel: [_ w208 _ _ _ _] -> w13
    tunnel: [_ w197 _ _ _ _] -> w12
    tunnel: [w44 _ _ _ _ _] -> w8
    tunnel: w7 -> [w45 _ _ _ _ _]
    tunnel: w6 -> [_ _ _ _ w381 _]
    tunnel: [_ _ _ _ w380 _] -> w5
    tunnel: w4 -> [w28 _ _ _ _ _]
    tunnel: [w26 _ _ _ _ _] -> w3
    frame #0 {
      n4 = Strip Path(path=w70) -> (name=w27:string)  [unwired: 1 out]
      "Procedure Name" <- w27
      n5 = Concatenate Strings(w27, "_pb4") -> (w94:string)
      n6 = Concatenate Strings(w27, "_rmp4") -> (w92:string)
      n7 = Concatenate Strings(w27, "_freq4") -> (w59:string)
      n8 = Concatenate Strings(w27, "_DDS4") -> (w42:string)
      n9 = Build Path(base path=w70, name or relative path="master") -> (appended path=w25:path)
      n10 = Build Path(base path=w25, name or relative path=w94) -> (appended path=w68:path)
      n11 = Build Path(base path=w25, name or relative path=w92) -> (appended path=w67:path)
      n12 = Build Path(base path=w25, name or relative path=w59) -> (appended path=w48:path)
      n13 = Build Path(base path=w25, name or relative path=w42) -> (appended path=w31:path)
      n14 = call <vilib>:"Open_Create_Replace File.vi"("file path"=w68) -> ("error out"=w83:errorcluster, "refnum"=w90:refnum<file>)  [unwired: 5 in, 4 out]
      n15 = call <vilib>:"Open_Create_Replace File.vi"("file path"=w67) -> ("error out"=w72:errorcluster, "refnum"=w79:refnum<file>)  [unwired: 5 in, 4 out]
      n16 = call <vilib>:"Open_Create_Replace File.vi"("file path"=w48) -> ("error out"=w50:errorcluster, "refnum"=w57:refnum<file>)  [unwired: 5 in, 4 out]
      n17 = call <vilib>:"Open_Create_Replace File.vi"("file path"=w31) -> ("error out"=w33:errorcluster, "refnum"=w40:refnum<file>)  [unwired: 5 in, 4 out]
      n18 = Get File Size(file=w90, error in=w83) -> (refnum out=w89:refnum<file>, size (in bytes)=w87:i64, 0:w82:errorcluster)
      n19 = Get File Size(file=w79, error in=w72) -> (refnum out=w78:refnum<file>, size (in bytes)=w76:i64, 0:w71:errorcluster)
      n20 = Get File Size(file=w57, error in=w50) -> (refnum out=w56:refnum<file>, size (in bytes)=w54:i64, 0:w49:errorcluster)
      n21 = Get File Size(file=w40, error in=w33) -> (refnum out=w39:refnum<file>, size (in bytes)=w37:i64, 0:w32:errorcluster)
      n22 = Unbundle By Name(w71) -> ("status"=w73:bool)
      n23 = Unbundle By Name(w49) -> ("status"=w51:bool)
      n24 = Unbundle By Name(w32) -> ("status"=w34:bool)
      n25 = Unbundle By Name(w82) -> ("status"=w84:bool)
      n26 = To Long Integer(number=w87) -> (32bit integer=w88:i32)
      n27 = To Long Integer(number=w76) -> (32bit integer=w77:i32)
      n28 = To Long Integer(number=w54) -> (32bit integer=w55:i32)
      n29 = To Long Integer(number=w37) -> (32bit integer=w38:i32)
      n30 = Equal To 0?(x=w88) -> (x = 0?=w85:bool)
      n31 = Equal To 0?(x=w77) -> (x = 0?=w74:bool)
      n32 = Equal To 0?(x=w55) -> (x = 0?=w52:bool)
      n33 = Equal To 0?(x=w38) -> (x = 0?=w35:bool)
      n34 = Index Array(array=w61, index=0) -> (element=w62:T10)
      n35 = Index Array(array=w45, index=0) -> (element=w46:T11)
      n36 = Index Array(array=w28, index=0) -> (element=w29:T11)
      n37 = Index Array(array=w65, index=0) -> (element=w64:T12)
      n38 = Or(x=w85, y=w84) -> (x .or. y?=w86:bool)
      n39 = Or(x=w74, y=w73) -> (x .or. y?=w75:bool)
      n40 = Or(x=w52, y=w51) -> (x .or. y?=w53:bool)
      n41 = Or(x=w35, y=w34) -> (x .or. y?=w36:bool)
      n42 = case shown="False" w86 {
        tunnel: [w171 w188] -> w91
        tunnel: w64 -> [w170 w186]
        tunnel: w89 -> [w169 w188]
        tunnel: [w168 w187] -> w81
        tunnel: w88 -> [w167 _]
        frame False {
          # "Read out each element from the data file"
          n43 = while {
            tunnel: [w182] -> w168 mode=indexing
            tunnel: w170 -> [w181]
            shift-right: [w183] -> w171
            shift-left: w169 -> [w184]
            tunnel: w167 -> [w180]
            shift-right: [w179] -> _
            shift-left: 0 -> [w178]
            stop <- w175 stop-if-true
            n44 = Read from Binary File(5:w181, 11:w184) -> (0:w173:errorcluster, 2:w182:T12, 3:w174:refnum<file>)  [unwired: 1 in, 4 out]
            n45 = Get File Position(4:w173, 7:w174) -> (2:w172:i64, 3:w183:refnum<file>)  [unwired: 1 out]
            n46 = To Long Integer(number=w172) -> (32bit integer=w179:i32)
            n47 = Greater Or Equal?(x=w179, y=w180) -> (x >= y?=w176:bool)
            n48 = Equal?(x=w179, y=w178) -> (x = y?=w177:bool)
            n49 = Or(x=w176, y=w177) -> (x .or. y?=w175:bool)
          }
        }
        frame True {
          n50 = Initialize Array(w186, 0) -> (w187:T3)
        }
      }
      n51 = case shown="False" w75 {
        tunnel: [w148 w165] -> w80
        tunnel: w62 -> [w147 w163]
        tunnel: w78 -> [w146 w165]
        tunnel: [w145 w164] -> w69
        tunnel: w77 -> [w144 _]
        frame False {
          # "Read out each element from the data file"
          n52 = while {
            tunnel: [w159] -> w145 mode=indexing
            tunnel: w147 -> [w158]
            shift-right: [w160] -> w148
            shift-left: w146 -> [w161]
            tunnel: w144 -> [w157]
            shift-right: [w156] -> _
            shift-left: 0 -> [w155]
            stop <- w152 stop-if-true
            n53 = Read from Binary File(5:w158, 11:w161) -> (0:w150:errorcluster, 2:w159:T10, 3:w151:refnum<file>)  [unwired: 1 in, 4 out]
            n54 = Get File Position(4:w150, 7:w151) -> (2:w149:i64, 3:w160:refnum<file>)  [unwired: 1 out]
            n55 = To Long Integer(number=w149) -> (32bit integer=w156:i32)
            n56 = Greater Or Equal?(x=w156, y=w157) -> (x >= y?=w153:bool)
            n57 = Equal?(x=w156, y=w155) -> (x = y?=w154:bool)
            n58 = Or(x=w153, y=w154) -> (x .or. y?=w152:bool)
          }
        }
        frame True {
          n59 = Initialize Array(w163, 0) -> (w164:T4)
        }
      }
      n60 = case shown="False" w53 {
        tunnel: [w125 w142] -> w58
        tunnel: w46 -> [w124 w140]
        tunnel: w56 -> [w123 w142]
        tunnel: [w122 w141] -> w44
        tunnel: w55 -> [w121 _]
        frame False {
          # "Read out each element from the data file"
          n61 = while {
            tunnel: [w136] -> w122 mode=indexing
            tunnel: w124 -> [w135]
            shift-right: [w137] -> w125
            shift-left: w123 -> [w138]
            tunnel: w121 -> [w134]
            shift-right: [w133] -> _
            shift-left: 0 -> [w132]
            stop <- w129 stop-if-true
            n62 = Read from Binary File(5:w135, 11:w138) -> (0:w127:errorcluster, 2:w136:T11, 3:w128:refnum<file>)  [unwired: 1 in, 4 out]
            n63 = Get File Position(4:w127, 7:w128) -> (2:w126:i64, 3:w137:refnum<file>)  [unwired: 1 out]
            n64 = To Long Integer(number=w126) -> (32bit integer=w133:i32)
            n65 = Greater Or Equal?(x=w133, y=w134) -> (x >= y?=w130:bool)
            n66 = Equal?(x=w133, y=w132) -> (x = y?=w131:bool)
            n67 = Or(x=w130, y=w131) -> (x .or. y?=w129:bool)
          }
        }
        frame True {
          n68 = Initialize Array(w140, 0) -> (w141:T5)
        }
      }
      n69 = case shown="False" w36 {
        tunnel: [w102 w119] -> w41
        tunnel: w29 -> [w101 w117]
        tunnel: w39 -> [w100 w119]
        tunnel: [w99 w118] -> w26
        tunnel: w38 -> [w98 _]
        frame False {
          # "Read out each element from the data file"
          n70 = while {
            tunnel: [w113] -> w99 mode=indexing
            tunnel: w101 -> [w112]
            shift-right: [w114] -> w102
            shift-left: w100 -> [w115]
            tunnel: w98 -> [w111]
            shift-right: [w110] -> _
            shift-left: 0 -> [w109]
            stop <- w106 stop-if-true
            n71 = Read from Binary File(5:w112, 11:w115) -> (0:w104:errorcluster, 2:w113:T11, 3:w105:refnum<file>)  [unwired: 1 in, 4 out]
            n72 = Get File Position(4:w104, 7:w105) -> (2:w103:i64, 3:w114:refnum<file>)  [unwired: 1 out]
            n73 = To Long Integer(number=w103) -> (32bit integer=w110:i32)
            n74 = Greater Or Equal?(x=w110, y=w111) -> (x >= y?=w107:bool)
            n75 = Equal?(x=w110, y=w109) -> (x = y?=w108:bool)
            n76 = Or(x=w107, y=w108) -> (x .or. y?=w106:bool)
          }
        }
        frame True {
          n77 = Initialize Array(w117, 0) -> (w118:T5)
        }
      }
      n78 = Close File(refnum=w80) -> ()  [unwired: 1 in, 2 out]
      n79 = Close File(refnum=w58) -> ()  [unwired: 1 in, 2 out]
      n80 = Close File(refnum=w41) -> ()  [unwired: 1 in, 2 out]
      n81 = Close File(refnum=w91) -> ()  [unwired: 1 in, 2 out]
    }
    frame #1 {
      n82 = Strip Path(path=w209) -> (name=w220:string)  [unwired: 1 out]
      n83 = Concatenate Strings(w220, "_pb4") -> (w224:string)
      n84 = Concatenate Strings(w220, "_rmp4") -> (w222:string)
      n85 = Build Path(base path=w209, name or relative path="slave") -> (appended path=w221:path)
      n86 = Build Path(base path=w221, name or relative path=w224) -> (appended path=w196:path)
      n87 = Build Path(base path=w221, name or relative path=w222) -> (appended path=w195:path)
      n88 = call <vilib>:"Open_Create_Replace File.vi"("file path"=w196) -> ("error out"=w211:errorcluster, "refnum"=w218:refnum<file>)  [unwired: 5 in, 4 out]
      n89 = call <vilib>:"Open_Create_Replace File.vi"("file path"=w195) -> ("error out"=w199:errorcluster, "refnum"=w206:refnum<file>)  [unwired: 5 in, 4 out]
      n90 = Get File Size(file=w218, error in=w211) -> (refnum out=w217:refnum<file>, size (in bytes)=w215:i64, 0:w210:errorcluster)
      n91 = Get File Size(file=w206, error in=w199) -> (refnum out=w205:refnum<file>, size (in bytes)=w203:i64, 0:w198:errorcluster)
      n92 = Unbundle By Name(w210) -> ("status"=w212:bool)
      n93 = Unbundle By Name(w198) -> ("status"=w200:bool)
      n94 = To Long Integer(number=w215) -> (32bit integer=w216:i32)
      n95 = To Long Integer(number=w203) -> (32bit integer=w204:i32)
      n96 = Equal To 0?(x=w216) -> (x = 0?=w213:bool)
      n97 = Equal To 0?(x=w204) -> (x = 0?=w201:bool)
      n98 = Index Array(array=w192, index=0) -> (element=w193:T12)
      n99 = Index Array(array=w189, index=0) -> (element=w190:T10)
      n100 = Or(x=w213, y=w212) -> (x .or. y?=w214:bool)
      n101 = Or(x=w201, y=w200) -> (x .or. y?=w202:bool)
      n102 = case shown="False" w214 {
        tunnel: [w255 w272] -> w219
        tunnel: w193 -> [w254 w270]
        tunnel: w217 -> [w253 w272]
        tunnel: [w252 w271] -> w208
        tunnel: w216 -> [w251 _]
        frame False {
          # "Read out each element from the data file"
          n103 = while {
            tunnel: [w266] -> w252 mode=indexing
            tunnel: w254 -> [w265]
            shift-right: [w267] -> w255
            shift-left: w253 -> [w268]
            tunnel: w251 -> [w264]
            shift-right: [w263] -> _
            shift-left: 0 -> [w262]
            stop <- w259 stop-if-true
            n104 = Read from Binary File(5:w265, 11:w268) -> (0:w257:errorcluster, 2:w266:T12, 3:w258:refnum<file>)  [unwired: 1 in, 4 out]
            n105 = Get File Position(4:w257, 7:w258) -> (2:w256:i64, 3:w267:refnum<file>)  [unwired: 1 out]
            n106 = To Long Integer(number=w256) -> (32bit integer=w263:i32)
            n107 = Greater Or Equal?(x=w263, y=w264) -> (x >= y?=w260:bool)
            n108 = Equal?(x=w263, y=w262) -> (x = y?=w261:bool)
            n109 = Or(x=w260, y=w261) -> (x .or. y?=w259:bool)
          }
        }
        frame True {
          n110 = Initialize Array(w270, 0) -> (w271:T3)
        }
      }
      n111 = case shown="False" w202 {
        tunnel: [w232 w249] -> w207
        tunnel: w190 -> [w231 w247]
        tunnel: w205 -> [w230 w249]
        tunnel: [w229 w248] -> w197
        tunnel: w204 -> [w228 _]
        frame False {
          # "Read out each element from the data file"
          n112 = while {
            tunnel: [w243] -> w229 mode=indexing
            tunnel: w231 -> [w242]
            shift-right: [w244] -> w232
            shift-left: w230 -> [w245]
            tunnel: w228 -> [w241]
            shift-right: [w240] -> _
            shift-left: 0 -> [w239]
            stop <- w236 stop-if-true
            n113 = Read from Binary File(5:w242, 11:w245) -> (0:w234:errorcluster, 2:w243:T10, 3:w235:refnum<file>)  [unwired: 1 in, 4 out]
            n114 = Get File Position(4:w234, 7:w235) -> (2:w233:i64, 3:w244:refnum<file>)  [unwired: 1 out]
            n115 = To Long Integer(number=w233) -> (32bit integer=w240:i32)
            n116 = Greater Or Equal?(x=w240, y=w241) -> (x >= y?=w237:bool)
            n117 = Equal?(x=w240, y=w239) -> (x = y?=w238:bool)
            n118 = Or(x=w237, y=w238) -> (x .or. y?=w236:bool)
          }
        }
        frame True {
          n119 = Initialize Array(w247, 0) -> (w248:T4)
        }
      }
      n120 = Close File(refnum=w219) -> ()  [unwired: 1 in, 2 out]
      n121 = Close File(refnum=w207) -> ()  [unwired: 1 in, 2 out]
    }
    frame #2 {
      n122 = local read "Procedure Name"() -> (w275:string)
      n123 = Concatenate Strings(w275, "_evp4") -> (w290:string)
      n124 = Build Path(base path=w276, name or relative path=w290) -> (appended path=w279:path)
      n125 = call <vilib>:"Open_Create_Replace File.vi"("file path"=w279) -> ("error out"=w281:errorcluster, "refnum"=w288:refnum<file>)  [unwired: 5 in, 4 out]
      n126 = Get File Size(file=w288, error in=w281) -> (refnum out=w287:refnum<file>, size (in bytes)=w285:i64, 0:w280:errorcluster)
      n127 = Unbundle By Name(w280) -> ("status"=w282:bool)
      n128 = To Long Integer(number=w285) -> (32bit integer=w286:i32)
      n129 = Equal To 0?(x=w286) -> (x = 0?=w283:bool)
      n130 = Index Array(array=w278, index=0) -> (element=w277:T13)
      n131 = Or(x=w283, y=w282) -> (x .or. y?=w284:bool)
      n132 = case shown="False" w284 {
        tunnel: [w297 w314] -> w289
        tunnel: w277 -> [w296 w311]
        tunnel: w287 -> [w295 w314]
        tunnel: [w294 w313] -> w273
        tunnel: w286 -> [w293 _]
        frame False {
          # "Read out each element from the data file"
          n133 = while {
            tunnel: [w308] -> w294 mode=indexing
            tunnel: w296 -> [w307]
            shift-right: [w309] -> w297
            shift-left: w295 -> [w310]
            tunnel: w293 -> [w306]
            shift-right: [w305] -> _
            shift-left: 0 -> [w304]
            stop <- w301 stop-if-true
            n134 = Read from Binary File(5:w307, 11:w310) -> (0:w299:errorcluster, 2:w308:T13, 3:w300:refnum<file>)  [unwired: 1 in, 4 out]
            n135 = Get File Position(4:w299, 7:w300) -> (2:w298:i64, 3:w309:refnum<file>)  [unwired: 1 out]
            n136 = To Long Integer(number=w298) -> (32bit integer=w305:i32)
            n137 = Greater Or Equal?(x=w305, y=w306) -> (x >= y?=w302:bool)
            n138 = Equal?(x=w305, y=w304) -> (x = y?=w303:bool)
            n139 = Or(x=w302, y=w303) -> (x .or. y?=w301:bool)
          }
        }
        frame True {
          n140 = Initialize Array(w311, 0) -> (w313:T6)
        }
      }
      n141 = Close File(refnum=w289) -> ()  [unwired: 1 in, 2 out]
    }
    frame #3 {
      n142 = local read "Procedure Name"() -> (w333:string)
      n143 = Concatenate Strings(w333, "_seq4") -> (w330:string)
      n144 = Build Path(base path=w319, name or relative path=w330) -> (appended path=w334:path)
      n145 = call <vilib>:"Open_Create_Replace File.vi"("file path"=w334) -> ("error out"=w321:errorcluster, "refnum"=w329:refnum<file>)  [unwired: 5 in, 4 out]
      n146 = Get File Size(file=w329, error in=w321) -> (refnum out=w328:refnum<file>, size (in bytes)=w325:i64, 0:w320:errorcluster)
      n147 = Unbundle By Name(w320) -> ("status"=w322:bool)
      n148 = To Long Integer(number=w325) -> (32bit integer=w326:i32)
      n149 = Equal To 0?(x=w326) -> (x = 0?=w323:bool)
      n150 = Index Array(array=w316, index=0) -> (element=w317:T14)
      n151 = Or(x=w323, y=w322) -> (x .or. y?=w324:bool)
      n152 = case shown="False" w324 {
        tunnel: [w350 w379] -> w332
        tunnel: w317 -> [w336 w377]
        tunnel: w328 -> [w349 w379]
        tunnel: [w335 w376] -> w327
        tunnel: w326 -> [w348 _]
        tunnel: [w346 errorcluster[] []] -> w315
        frame False {
          # "The Bundles/Unbundles fix a data type mismatch \nbetween this version and version 4.10 DDS"
          # "Read out each element from the data file"
          n153 = Unbundle By Name(w336) -> ("Start"=w345:dbl, "End"=w344:dbl, "Sequenced Data"=w343:dbl[], "Inform\nIgor?"=w342:bool, "Computed Step Size"=w341:dbl, "Procedure Variable"=w340:string, "Default"=w339:dbl)  [unwired: 1 out]
          n154 = Bundle By Name(cluster=T9 {"Start"=0.0, "End"=0.0, "Sequenced Data"=[], "Inform\nIgor?"=FALSE, "Computed Step Size"=0.0, "Procedure Variable"="", "Default"=0.0} ("Sequencing Info"), "Start"=w345, "End"=w344, "Sequenced Data"=w343, "Inform\nIgor?"=w342, "Computed Step Size"=w341, "Procedure Variable"=w340, "Default"=w339) -> (w337:T9)
          n155 = while {
            tunnel: w337 -> [w372]
            shift-right: [w373] -> w350
            shift-left: w349 -> [w374]
            tunnel: w348 -> [w371]
            shift-right: [w370] -> _
            shift-left: 0 -> [w369]
            tunnel: [w362] -> w346 mode=indexing
            tunnel: w336 -> [w361]
            tunnel: [w352] -> w335 mode=indexing
            stop <- w366 stop-if-true
            n156 = Read from Binary File(5:w372, 11:w374) -> (0:w364:errorcluster, 2:w360:T9, 3:w365:refnum<file>)  [unwired: 1 in, 4 out]
            n157 = Unbundle By Name(w360) -> ("Start"=w359:dbl, "End"=w358:dbl, "Sequenced Data"=w357:dbl[], "Inform\nIgor?"=w356:bool, "Computed Step Size"=w355:dbl, "Procedure Variable"=w354:string, "Default"=w353:dbl)
            n158 = Get File Position(4:w364, 7:w365) -> (0:w362:errorcluster, 2:w363:i64, 3:w373:refnum<file>)
            n159 = To Long Integer(number=w363) -> (32bit integer=w370:i32)
            n160 = Greater Or Equal?(x=w370, y=w371) -> (x >= y?=w367:bool)
            n161 = Equal?(x=w370, y=w369) -> (x = y?=w368:bool)
            n162 = Or(x=w367, y=w368) -> (x .or. y?=w366:bool)
            n163 = Bundle By Name(cluster=w361, "Start"=w359, "End"=w358, "Sequenced Data"=w357, "Inform\nIgor?"=w356, "Computed Step Size"=w355, "Procedure Variable"=w354, "Default"=w353, "Steps"=10) -> (w352:T14)
          }
        }
        frame True {
          n164 = Initialize Array(w377, 0) -> (w376:T7)
        }
      }
      "Array" <- w315
      n165 = Close File(refnum=w332) -> ()  [unwired: 1 in, 2 out]
    }
    frame #4 {
      n166 = local read "Procedure Name"() -> (w397:string)
      n167 = Concatenate Strings(w397, "_var4") -> (w394:string)
      n168 = Build Path(base path=w384, name or relative path=w394) -> (appended path=w398:path)
      n169 = call <vilib>:"Open_Create_Replace File.vi"("file path"=w398) -> ("error out"=w386:errorcluster, "refnum"=w393:refnum<file>)  [unwired: 5 in, 4 out]
      n170 = Get File Size(file=w393, error in=w386) -> (refnum out=w392:refnum<file>, size (in bytes)=w390:i64, 0:w385:errorcluster)
      n171 = Unbundle By Name(w385) -> ("status"=w387:bool)
      n172 = To Long Integer(number=w390) -> (32bit integer=w391:i32)
      n173 = Equal To 0?(x=w391) -> (x = 0?=w388:bool)
      n174 = Index Array(array=w381, index=0) -> (element=w382:T1)
      n175 = Or(x=w388, y=w387) -> (x .or. y?=w389:bool)
      n176 = case shown="True" w389 {
        tunnel: [w404 w421] -> w396
        tunnel: w382 -> [w403 w419]
        tunnel: w392 -> [w402 w421]
        tunnel: [w401 w418] -> w380
        tunnel: w391 -> [w400 _]
        frame False {
          # "Read out each element from the data file"
          n177 = while {
            tunnel: [w415] -> w401 mode=indexing
            tunnel: w403 -> [w414]
            shift-right: [w416] -> w404
            shift-left: w402 -> [w417]
            tunnel: w400 -> [w413]
            shift-right: [w412] -> _
            shift-left: 0 -> [w411]
            stop <- w408 stop-if-true
            n178 = Read from Binary File(5:w414, 11:w417) -> (0:w406:errorcluster, 2:w415:T1, 3:w407:refnum<file>)  [unwired: 1 in, 4 out]
            n179 = Get File Position(4:w406, 7:w407) -> (2:w405:i64, 3:w416:refnum<file>)  [unwired: 1 out]
            n180 = To Long Integer(number=w405) -> (32bit integer=w412:i32)
            n181 = Greater Or Equal?(x=w412, y=w413) -> (x >= y?=w409:bool)
            n182 = Equal?(x=w412, y=w411) -> (x = y?=w410:bool)
            n183 = Or(x=w409, y=w410) -> (x .or. y?=w408:bool)
          }
        }
        frame True {
          n184 = Initialize Array(w419, 0) -> (w418:T1[])
        }
      }
      n185 = Close File(refnum=w396) -> ()  [unwired: 1 in, 2 out]
    }
    frame #5 {
      n186 = local read "Procedure Name"() -> (w439:string)
      n187 = Concatenate Strings(w439, "_srs4") -> (w437:string)
      n188 = Build Path(base path=w425, name or relative path=w437) -> (appended path=w440:path)
      n189 = call <vilib>:"Open_Create_Replace File.vi"("file path"=w440) -> ("error out"=w426:errorcluster, "refnum"=w433:refnum<file>)  [unwired: 5 in, 4 out]
      n190 = Get File Size(file=w433, error in=w426) -> (refnum out=w436:refnum<file>, size (in bytes)=w432:i64, 0:w427:errorcluster)
      n191 = Unbundle By Name(w427) -> ("status"=w428:bool)
      n192 = To Long Integer(number=w432) -> (32bit integer=w431:i32)
      n193 = Equal To 0?(x=w431) -> (x = 0?=w429:bool)
      n194 = Index Array(array=w422, index=0) -> (element=w423:T15)
      n195 = Or(x=w429, y=w428) -> (x .or. y?=w430:bool)
      n196 = case shown="False" w430 {
        tunnel: w436 -> [w445 w459]
        tunnel: [w444 w459] -> w435
        tunnel: [w443 w456] -> w434
        tunnel: w423 -> [w442 w457]
        tunnel: w431 -> [w441 _]
        frame False {
          # "Read out each element from the data file"
          n197 = while {
            tunnel: [w453] -> w443 mode=indexing
            tunnel: w442 -> [w452]
            shift-right: [w454] -> w444
            shift-left: w445 -> [w455]
            tunnel: w441 -> [w451]
            stop <- w449 stop-if-true
            n198 = Read from Binary File(5:w452, 11:w455) -> (0:w447:errorcluster, 2:w453:T15, 3:w448:refnum<file>)  [unwired: 1 in, 4 out]
            n199 = Get File Position(4:w447, 7:w448) -> (2:w446:i64, 3:w454:refnum<file>)  [unwired: 1 out]
            n200 = To Long Integer(number=w446) -> (32bit integer=w450:i32)
            n201 = Greater Or Equal?(x=w450, y=w451) -> (x >= y?=w449:bool)
          }
        }
        frame True {
          n202 = Initialize Array(w457, 0) -> (w456:T8)
        }
      }
      n203 = Close File(refnum=w435) -> ()  [unwired: 1 in, 2 out]
    }
  }
  n204 = local read "Paramaters"() -> (w24:T2)
  n205 = Bundle By Name(cluster=w24, "Master PB Staging List"=w16, "Master AO Ramp List"=w14, "Master Novatech Ramp List"=w8, "Novatech Ramps"=w11, "Sequencing Info"=w10, "SRS Ramps"=w9, "Slave PB Staging List"=w13, "Slave AO Ramp List"=w12, "Static Variables"=w5, "DDS Ramp List"=w3) -> (→"Paramaters":T2)
